vi "RegisterMat_Array1D-2DPoint-DBL.vi"(8 "error in":errorcluster, 11 "Array in":T1[](array[typedef])) -> (0 "error out":errorcluster, 3 "Image":u8, 4 "AdressOrData":T1[](array[typedef]), 6 "Mat":T2)   [LabVIEW 2020, in "OpenLvVision_OpenCv.lvlib"]
doc: "Register mat for dll.\nNo malleable to breake vi inlining!"
uses:
  OpenLvVision_OpenCv.lvlib
  TypeDef/MatInfo.ctl
  TypeDef/LvDatatype.ctl
  TypeDef/Point/2D_PointDBL.ctl
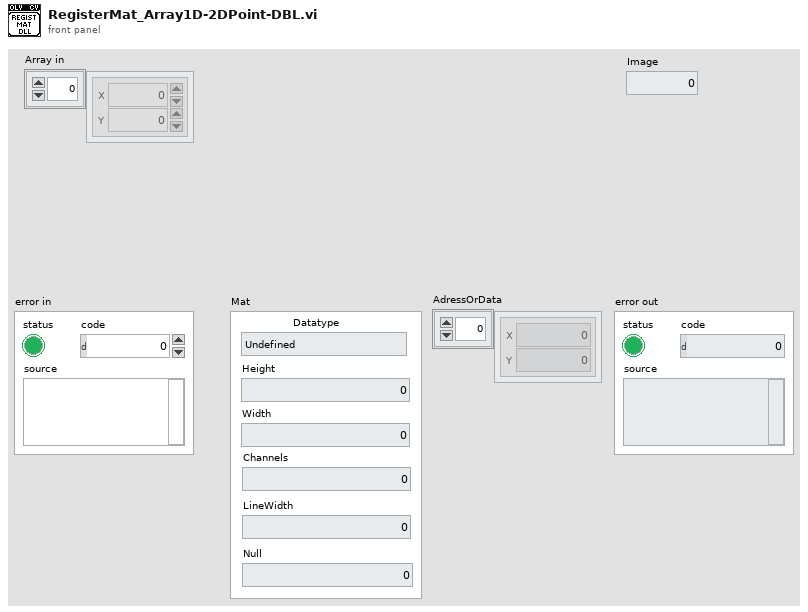
[diagram p1: front panel]
types:
  T1 = typedef "OpenLvVision_OpenCv.lvlib/2D_PointDBL.ctl" = cluster{"X":dbl, "Y":dbl}
  T2 = typedef "OpenLvVision_OpenCv.lvlib/MatInfo.ctl" = cluster{"Datatype":T3, "Height":i32, "Width":i32, "Channels":i32, "LineWidth":i32, "Null":u8}
  T3 = typedef "OpenLvVision_OpenCv.lvlib/LvDatatype.ctl" = enum32{"Undefined", "U8", "I8", "U16", "I16", "U32_Color", "I32", "U64_Color", "I64", "SGL", "DBL", "Complex SGL", "Complex DBL", "Array 1D U8", "Array 1D I8", "Array 1D U16", "Array 1D I16", "Array 1D U32_Color", "Array 1D I32", "Array 1D U64_Color", "Array 1D I64", "Array 1D SGL", "Array 1D DBL", "Array 1D Complex SGL", "Array 1D Complex DBL", "Array 2D U8", "Array 2D I8", "Array 2D U16", "Array 2D I16", "Array 2D U32", "Array 2D U32_Color", "Array 2D I32", "Array 2D U64", "Array 2D U64_Color", "Array 2D I64", "Array 2D SGL", "Array 2D DBL", "Array 2D Complex SGL", "Array 2D Complex DBL", "Image Mono U8", "Image Mono U16", "Image Mono I16", "Image Mono SGL", "Image Color U32", "Image Color U64", "ImageComplex Sgl", "Array1d_2dPointI32", "Array1d_2dPointSGL", "Array1d_2dPointDBL", "Array1d_3dPointI32", "Array1d_3dPointSGL", "Array1d_3dPointDBL", "Array1d_4dPointI32", "Array1d_4dPointSGL", "Array1d_4dPointDBL"}
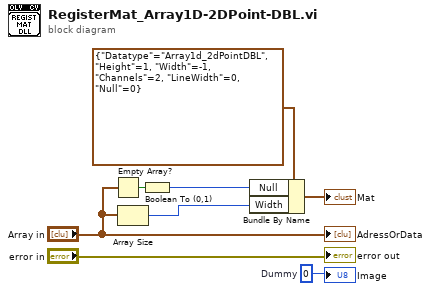
[diagram p0: block diagram]
diagram:
  w2 = u8 0  # Dummy
  n1 = Empty Array?(array="Array in") -> (empty?=w6:bool)
  n2 = Array Size(array="Array in") -> (size(s)=w7:i32)
  n3 = Boolean To (0,1)(Boolean=w6) -> (0, 1=w5:i16)
  n4 = Bundle By Name(cluster=T2 {"Datatype"=enum."Array1d_2dPointDBL", "Height"=1, "Width"=-1, "Channels"=2, "LineWidth"=0, "Null"=0} ("LvData"), "Null"=w5, "Width"=w7) -> (→"Mat":T2)
  "error out" <- "error in"
  "AdressOrData" <- "Array in"
  "Image" <- w2
